vi "Auto_Routine_DepositConeBalance.vi"(8 "error in (no error)":errorcluster, 11 "IsBlue?":bool) -> (0 "error out":errorcluster)   [LabVIEW 2020]
doc: "deposits cone, drives backwards, balances. Starts from 3rd node from non pickup edge. Determines is it is blue or red (by IsBlue?) then changes actions accordingly.\n\ninputs: \n--IsBlue?--Boolean--\n--ErrorIn--\noutputs:\n--ErrorOut--"
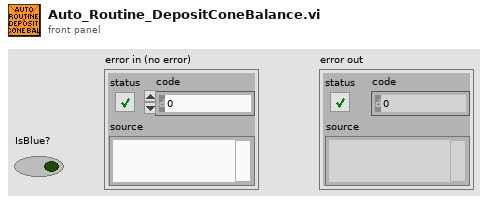
[diagram p1: front panel]
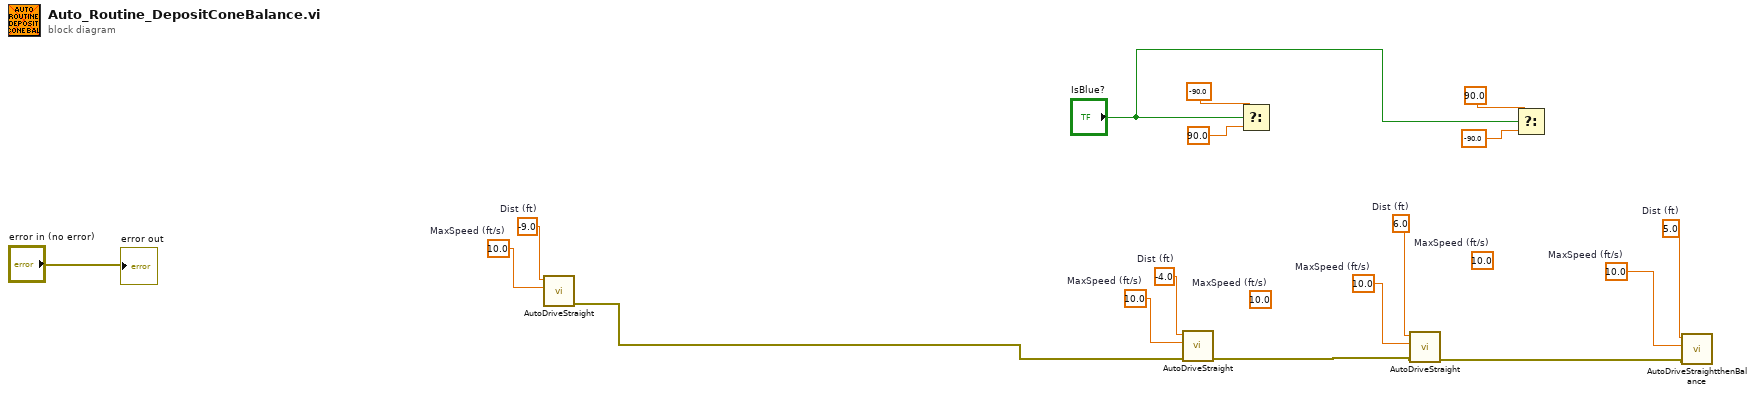
[diagram p0: block diagram]
diagram:
  w9 = 10.0  # MaxSpeed (ft/s)
  w10 = 5.0  # Dist (ft)
  (unwired) 10.0  # MaxSpeed (ft/s)
  w11 = 10.0  # MaxSpeed (ft/s)
  w12 = 6.0  # Dist (ft)
  (unwired) 10.0  # MaxSpeed (ft/s)
  w13 = -4.0  # Dist (ft)
  w14 = 10.0  # MaxSpeed (ft/s)
  w15 = -9.0  # Dist (ft)
  w16 = 10.0  # MaxSpeed (ft/s)
  n1 = call "AutoDriveStraight.vi"("MaxSpeed (ft/s)"=w16, "Dist (ft)"=w15) -> ("error out"=w3:errorcluster)  [unwired: 9 in]
  n2 = call "AutoDriveStraight.vi"("error in (no error)"=w3, "MaxSpeed (ft/s)"=w14, "Dist (ft)"=w13) -> ("error out"=w2:errorcluster)  [unwired: 8 in]
  n3 = Select(t=-90.0, s="IsBlue?", f=90.0) -> ()  [unwired: 1 out]
  n4 = call "AutoDriveStraight.vi"("error in (no error)"=w2, "MaxSpeed (ft/s)"=w11, "Dist (ft)"=w12) -> ("error out"=w1:errorcluster)  [unwired: 8 in]
  n5 = Select(t=90.0, s="IsBlue?", f=-90.0) -> ()  [unwired: 1 out]
  n6 = call "AutoDriveStraightthenBalance.vi"("error in (no error)"=w1, "MaxSpeed (ft/s)"=w9, "Dist (ft)"=w10) -> ()  [unwired: 8 in, 1 out]
  "error out" <- "error in (no error)"
